vi "QueueHandler.vi"(6 "CMD":enum16{"Init", "GetRef", "Distroy"}(ring)=enum."GetRef", 8 "Error In":errorcluster) -> (0 "Error Out":errorcluster, 2 "UI":refnum<queue>, 3 "Win":refnum<queue>)   [LabVIEW 2025]
uses:
  Controls/Queue_Data.ctl
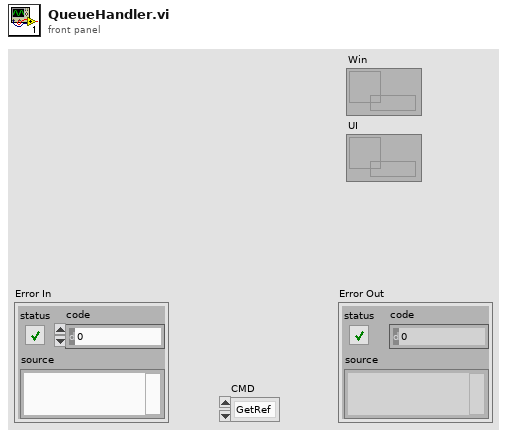
[diagram p1: front panel]
types:
  T1 = typedef "Queue_Data.ctl" = cluster{"CMD":string, "Data":variant}
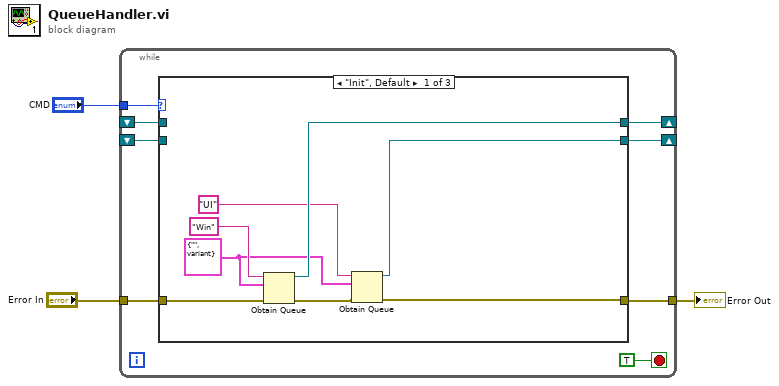
[diagram p0: block diagram]
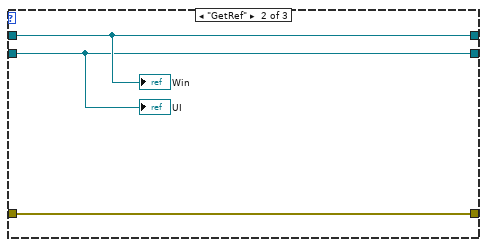
[diagram p2: hidden frame]
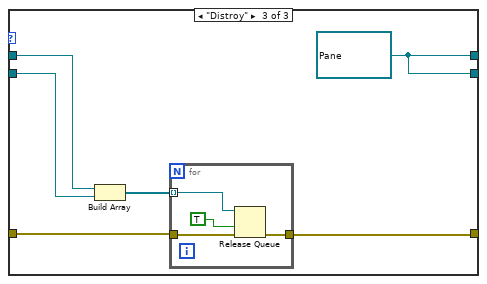
[diagram p3: hidden frame]
diagram:
  n1 = while {
    tunnel: "CMD" -> [w10]
    tunnel: "Error In" -> [w9]
    tunnel: [w8] -> w1
    shift-right: [w7] -> _
    shift-left: _ -> [w6]
    shift-right: [w5] -> _
    shift-left: _ -> [w4]
    stop <- TRUE stop-if-true
    n2 = case shown="\"Init\", Default" w10 {
      tunnel: w9 -> [w18 w22 w28]
      tunnel: [w15 w22 w27] -> w8
      tunnel: [w17 w21 w23] -> w7
      tunnel: w6 -> [_ w21 w26]
      tunnel: [w12 w20 w23] -> w5
      tunnel: w4 -> [_ w20 w25]
      frame "Init", Default {
        w14 = T1 {"CMD"="", "Data"=variant}
        n3 = Obtain Queue(name (unnamed)="Win", element data type=w14, error in (no error)=w18) -> (queue out=w17:refnum<queue>, error out=w16:errorcluster)  [unwired: 2 in, 1 out]
        n4 = Obtain Queue(name (unnamed)="UI", element data type=w14, error in (no error)=w16) -> (queue out=w12:refnum<queue>, error out=w15:errorcluster)  [unwired: 2 in, 1 out]
      }
      frame "GetRef" {
        "Win" <- w21
        "UI" <- w20
      }
      frame "Distroy" {
        w23 = refnum<queue> refnum ("queue out")
        n5 = Build Array(w26, w25) -> (w24:refnum<queue>[])
        n6 = for {
          tunnel: w28 -> [w32]
          tunnel: [w30] -> w27
          tunnel: w24 -> [w29] mode=indexing
          n7 = Release Queue(queue=w29, force destroy? (F)=TRUE, error in (no error)=w32) -> (error out=w30:errorcluster)  [unwired: 2 out]
        }
      }
    }
  }
  "Error Out" <- w1
